vi "OffsetRect by Point and Rect.vi"(8 "错误输入":errorcluster, 10 "point":cluster{"x":i16, "y":i16} caption="点", 11 "rect":T1 caption="矩形") -> (0 "错误输出":errorcluster, 3 "offset rect":T1 caption="偏移矩形")   [LabVIEW 2012, in "Rect Tools.lvlib"]
uses:
  Rect Tools.lvlib
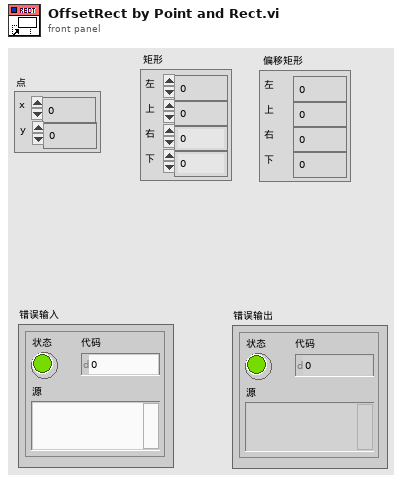
[diagram p1: front panel]
types:
  T1 = cluster{"left":i16, "top":i16, "right":i16, "bottom":i16}
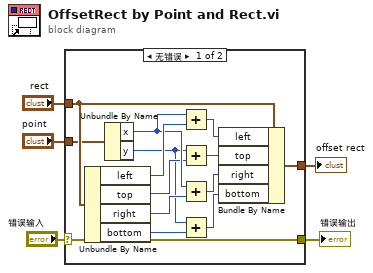
[diagram p0: block diagram]
diagram:
  n1 = case shown="无错误" "错误输入" {
    selector: "错误输入" -> [w9 w21]
    tunnel: [w9 w21] -> w4
    tunnel: "rect" -> [w8 w20]
    tunnel: [w7 w20] -> w2
    tunnel: "point" -> [w6 _]
    frame No Error {
      n2 = Unbundle By Name(w8) -> ("left"=w19:i16, "top"=w14:i16, "right"=w17:i16, "bottom"=w12:i16)
      n3 = Unbundle By Name(w6) -> ("x"=w16:i16, "y"=w13:i16)
      n4 = Add(x=w16, y=w19) -> (x+y=w18:i16)
      n5 = Add(x=w13, y=w14) -> (x+y=w10:i16)
      n6 = Add(x=w16, y=w17) -> (x+y=w15:i16)
      n7 = Add(x=w13, y=w12) -> (x+y=w11:i16)
      n8 = Bundle By Name(cluster=w8, "left"=w18, "top"=w10, "right"=w15, "bottom"=w11) -> (w7:T1)
    }
    frame Error {
    }
  }
  "错误输出" <- w4
  "offset rect" <- w2
